vi "ConfigureDataEventCreator.vi"(8 "error in (no error)":errorcluster) -> (0 "error out":errorcluster, 2 "valid configuration":bool, 3 "config":T1)   [LabVIEW 2017, in "CmsDataEventCreator.lvlib"]
uses:
  <vilib>/addons/InsightCM/Devices/Shared/Cms/CmsDataEventCreator/CmsDataEventCreator.lvlib
  <vilib>/addons/InsightCM/Devices/Shared/Cms/CmsDataEventCreator/controls/config.ctl
  <vilib>/addons/InsightCM/Devices/Shared/Cms/CmsDataEventCreator/controls/DataEventConfig.ctl
  <vilib>/addons/InsightCM/Devices/Shared/Cms/CmsDataEventCreator/controls/AcqParams.ctl
  <vilib>/addons/InsightCM/Devices/Shared/Common/DataAccumulator/controls/AccumulationSettings.ctl
  <vilib>/addons/InsightCM/Devices/Shared/Common/DataAccumulator/controls/accumulationType.ctl
  <vilib>/addons/InsightCM/Devices/Shared/Common/DVRBuffer/controls/BufferLocation.ctl
  <vilib>/addons/PointValueMap/controls/PointMap.ctl
  <vilib>/addons/InsightCM/Devices/Shared/Cms/CmsDataEventCreator/controls/GroupRegistry.ctl
  <vilib>/addons/InsightCM/Devices/Shared/Cms/CmsDataEventCreator/controls/DataSetRegistry.ctl
  <vilib>/addons/InsightCM/Devices/Shared/Common/DataEvent/controls/DataSetType.ctl
  <vilib>/addons/InsightCM/Devices/Shared/Common/DataEventCreator/controls/Registry_Trend.ctl
  <vilib>/addons/InsightCM/Devices/Shared/Common/DataEvent/controls/Event.ctl
  <vilib>/addons/InsightCM/MessageBus/Base/controls/DataEvent.ctl
  <vilib>/addons/InsightCM/MessageBus/Base/controls/KeyValuePair.ctl
  <vilib>/addons/InsightCM/Devices/Shared/Common/DataEvent/controls/DataSet.ctl
  <vilib>/addons/InsightCM/MessageBus/Base/controls/DataSetMetadata.ctl
  <vilib>/addons/InsightCM/MessageBus/Base/controls/TrendPoint.ctl
  <vilib>/addons/InsightCM/MessageBus/Base/controls/TrendAlarmUpdate.ctl
  <vilib>/addons/InsightCM/MessageBus/Base/controls/TrendAlarmTransition.ctl
  <vilib>/addons/InsightCM/Utilities/GlobalConfiguration/GlobalConfiguration.lvlib
  <vilib>/addons/PointValueMap/PointValueMap.lvlib
  <vilib>/addons/InsightCM/Devices/Shared/Common/DataEvent/DataEvent.lvlib
  <vilib>/addons/InsightCM/Devices/Shared/Common/DataEventCreator/DataEventCreator.lvlib
  <vilib>/addons/InsightCM/Utilities/PropertyHelpers/PropertyHelpers.lvlib
  <vilib>/addons/InsightCM/Devices/Shared/Common/DVRBuffer/DVRBuffer.lvlib
  <vilib>/addons/InsightCM/Devices/Shared/Common/DataAccumulator/DataAccumulator.lvlib
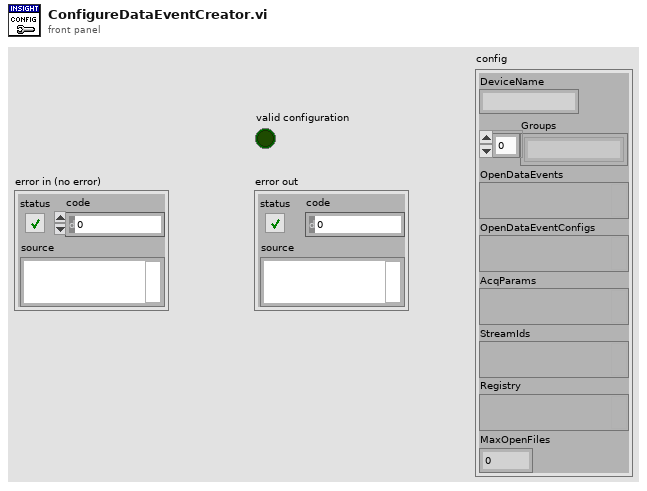
[diagram p1: front panel]
types:
  T1 = typedef "CmsDataEventCreator.lvlib/config.ctl" = cluster{"DeviceName":string, "Groups":string[], "OpenDataEvents":variant, "OpenDataEventConfigs":variant, "AcqParams":variant, "StreamIds":variant, "Registry":variant, "MaxOpenFiles":i32}
  T2 = typedef "SectionKeyValues.ctl" = cluster{"Section":string, "KeyValues":T3[]}
  T3 = typedef "KeyValuePair.ctl" = cluster{"Key":string, "Value":string}
  T4 = typedef "R2_Channel.ctl" = cluster{"Id":string, "DeviceId":string, "Name":string, "ChannelType":string, "HardwareKey":string, "HardwareChannel":string, "DataGroup":string, "Keywords":string[], "EquipmentIds":string[], "Properties":T3[], "Metrics":T5[], "AssetNodeId":string, "MeasType":string, "AssetName":string}
  T5 = typedef "Metric.ctl" = cluster{"Id":string, "Name":string, "Unit":string, "Properties":T3[], "MetricDefinitionInstanceId":string}
  T6 = typedef "R2_Device.ctl" = cluster{"Id":string, "Name":string, "DeviceType":string, "HardwareName":string, "IpAddress":string, "HardwareInfo":T3[], "ApplicationType":string, "ApplicationVersion":string, "EquipmentIds":string[], "ConfigurationVersion":string, "State":T7, "Properties":T3[], "DataGroups":T8[], "BurstModeTrigger":T12}
  T7 = typedef "DeviceState.ctl" = cluster{"Disabled":bool}
  T8 = typedef "R2_DataGroup.ctl" = cluster{"Name":string, "OperatingStates":T9[], "Properties":T3[], "EquipmentIds":string[], "AssetNodeId":string}
  T9 = typedef "OperatingState.ctl" = cluster{"Name":string, "Properties":T3[], "Triggers":T10[]}
  T10 = typedef "Trigger.ctl" = cluster{"Type":string, "Expression":string, "Conditions":T11[]}
  T11 = typedef "Condition.ctl" = cluster{"Source":string, "Type":string, "Operator":string, "CompareTo":string, "DwellSeconds":dbl}
  T12 = typedef "BurstModeTrigger.ctl" = cluster{"Trigger":T10, "SampleRate":string, "AcquisitionLength":string}
  T13 = typedef "DataEvent.lvlib/Event.ctl" = cluster{"DataEvent":T14, "DataSets":T15[], "TrendPoints":T17[], "Alarms":T18[]}
  T14 = typedef "DataEvent.ctl" = cluster{"Id":string, "AssetNodeId":string, "Timestamp":i64, "Props":T3[]}
  T15 = typedef "DataEvent.lvlib/DataSet.ctl" = cluster{"DataSetMetadata":T16, "Values":sgl[], "Values DVR":refnum<data-value>}
  T16 = typedef "DataSetMetadata.ctl" = cluster{"Id":string, "DataEventId":string, "AssetNodeId":string, "Type":string, "T0":i64, "Props":T3[]}
  T17 = typedef "TrendPoint.ctl" = cluster{"TrendPointId":string, "DataEventId":string, "Timestamp":i64, "Value":dbl, "Props":T3[]}
  T18 = typedef "TrendAlarmUpdate.ctl" = cluster{"RuleId":string, "Transition":T19}
  T19 = typedef "TrendAlarmTransition.ctl" = cluster{"At":i64, "Severity":i32, "Value":dbl, "Properties":T3[]}
  T20 = typedef "CmsDataEventCreator.lvlib/GroupRegistry.ctl" = cluster{"AssetNodeMap":variant, "DataSets":T21[], "Trends":T23[]}
  T21 = typedef "CmsDataEventCreator.lvlib/DataSetRegistry.ctl" = cluster{"ChannelName":string, "DataSetType":T22, "DoNotWriteToDB":bool, "ParentName":string, "CalculateOnServer":bool}
  T22 = typedef "DataEvent.lvlib/DataSetType.ctl" = enum16{"Waveform", "SpeedProfile", "ThermalImage", "EmsaSweep"}
  T23 = typedef "DataEventCreator.lvlib/Registry_Trend.ctl" = cluster{"TrendPointId":string, "DataSetName":string, "HighRate":bool, "Always Send":bool}
  T24 = typedef "CmsDataEventCreator.lvlib/DataEventConfig.ctl" = cluster{"AcqParams":T25, "OpState":string, "ExitOpState":bool, "Reason":string, "StreamId":string, "Map":T29, "DataSetIds":variant, "IncludeWaveforms":bool, "TrendPointsOnly":bool}
  T25 = typedef "CmsDataEventCreator.lvlib/AcqParams.ctl" = cluster{"Stream":bool, "PreTrigger":i32, "CollectOnEnter":bool, "Enter PreTrigger":i32, "Enter Length":dbl, "CollectOnExit":bool, "ContinuousData":bool, "Accumulation Settings":T26}
  T26 = typedef "DataAccumulator.lvlib/AccumulationSettings.ctl" = cluster{"Type":T27, "Length":dbl, "Max Time (sec)":dbl, "Start Block":T28, "Acquired (sec)":dbl, "Acquired (pulses)":i32, "Initial Pulse Offset":dbl, "Stop Block":T28, "LastBlockAdded":u32}
  T27 = typedef "DataAccumulator.lvlib/accumulationType.ctl" = enum16{"none", "seconds", "revolutions"}
  T28 = typedef "DVRBuffer.lvlib/BufferLocation.ctl" = cluster{"Block":u32, "Index":i32}
  T29 = typedef "PointValueMap.lvlib/PointMap.ctl" = refnum<data-value>
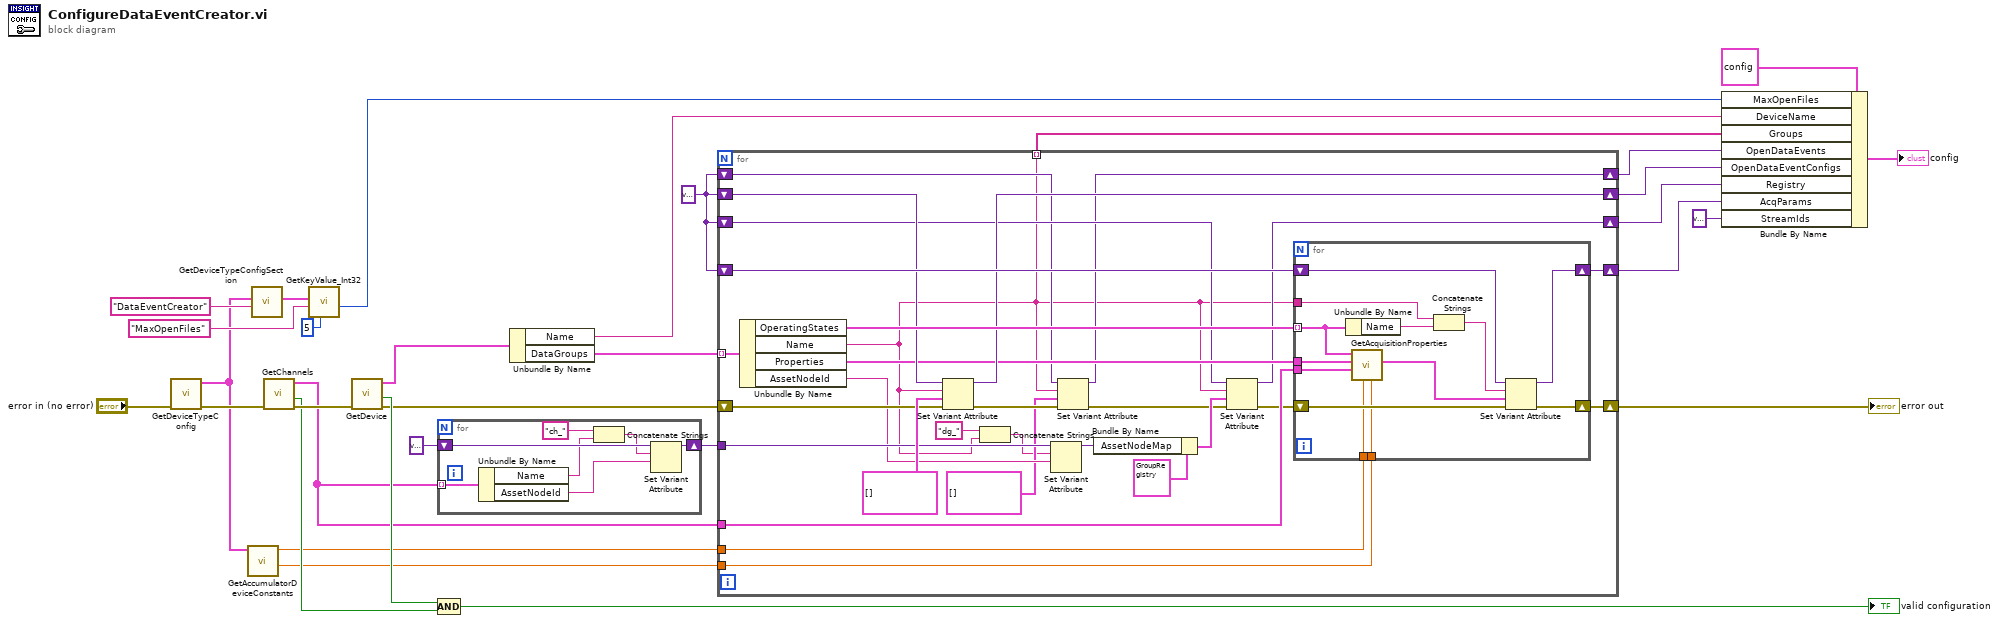
[diagram p0: block diagram]
diagram:
  w3 = variant
  n1 = call <vilib>:"GetDeviceTypeConfig.vi"("error in (no error)"="error in (no error)") -> ("error out"=w15:errorcluster, "key values"=w9:T2[])  [unwired: 8 in, 1 out]
  n2 = call <vilib>:"GetAccumulatorDeviceConstants.vi"("key values"=w9) -> ("default data block length (sec)"=w8:dbl, "max block (sec)"=w6:dbl)  [unwired: 6 in, 3 out]
  n3 = call <vilib>:"GetDeviceTypeConfigSection.vi"("key"="DataEventCreator", "key values"=w9) -> ("key value pairs out"=w13:T3[])  [unwired: 8 in, 1 out]
  n4 = call <vilib>:"GetChannels.vi"("error in (no error)"=w15) -> ("error out"=w23:errorcluster, "found"=w22:bool, "channels"=w18:T4[])  [unwired: 8 in]
  n5 = call <vilib>:"GetKeyValue_Int32.vi"("default"=5, "key"="MaxOpenFiles", "key value pairs"=w13) -> ("value"=w10:i32)  [unwired: 6 in, 2 out]
  n6 = call <vilib>:"GetDevice.vi"("error in (no error)"=w23) -> ("error out"=w20:errorcluster, "found"=w27:bool, "device configuration"=w30:T6)  [unwired: 8 in]
  n7 = for {
    shift-right: [w36] -> w17
    shift-left: variant -> [w37]
    tunnel: w18 -> [w38] mode=indexing
    n8 = Unbundle By Name(w38) -> ("Name"=w33:string, "AssetNodeId"=w35:string)
    n9 = Concatenate Strings("ch_" ("string"), w33) -> (w32:string)
    n10 = Set Variant Attribute(Variant=w37, name=w32, value=w35) -> (Variant out=w36:variant)  [unwired: 1 in, 2 out]
  }
  n11 = Compound Arithmetic op=AND(w27, w22) -> (→"valid configuration":bool)
  n12 = Unbundle By Name(w30) -> ("Name"=w24:string, "DataGroups"=w31:T8[])
  n13 = for {
    shift-right: [w56] -> w29
    shift-left: w20 -> [w57]
    tunnel: w31 -> [w66] mode=indexing
    shift-right: [w63] -> w25
    shift-left: w3 -> [w65]
    shift-right: [w61] -> w4
    shift-left: w3 -> [w62]
    tunnel: w18 -> [w58]
    shift-right: [w54] -> w5
    shift-left: w3 -> [w55]
    tunnel: w17 -> [w50]
    tunnel: w8 -> [w48]
    tunnel: w6 -> [w47]
    shift-right: [w43] -> w2
    shift-left: w3 -> [w44]
    tunnel: [w39] -> w1 mode=indexing
    n14 = Unbundle By Name(w66) -> ("OperatingStates"=w64:T9[], "Name"=w39:string, "Properties"=w59:T3[], "AssetNodeId"=w49:string)
    n15 = Set Variant Attribute(Variant=w62, name=w39, value=T24[] [], error in=w57) -> (Variant out=w61:variant, error out=w46:errorcluster)  [unwired: 1 out]
    n16 = Concatenate Strings("dg_" ("string"), w39) -> (w40:string)
    n17 = Set Variant Attribute(Variant=w50, name=w40, value=w49) -> (Variant out=w51:variant)  [unwired: 1 in, 2 out]
    n18 = Set Variant Attribute(Variant=w44, name=w39, value=T13[] [] ("data events"), error in=w46) -> (Variant out=w43:variant, error out=w45:errorcluster)  [unwired: 1 out]
    n19 = Bundle By Name(cluster=T20 {"AssetNodeMap"=variant, "DataSets"=[], "Trends"=[]} ("Data Group Registry"), "AssetNodeMap"=w51) -> (w52:T20)
    n20 = Set Variant Attribute(Variant=w55, name=w39, value=w52, error in=w45) -> (Variant out=w54:variant, error out=w56:errorcluster)  [unwired: 1 out]
    n21 = for {
      shift-right: [w69] -> _
      shift-left: w56 -> [w79]
      shift-right: [w77] -> w63
      shift-left: w65 -> [w78]
      tunnel: w39 -> [w75]
      tunnel: w64 -> [w73] mode=indexing
      tunnel: w59 -> [w72]
      tunnel: w58 -> [w71]
      tunnel: w48 -> [w67]
      tunnel: w47 -> [w68]
      n22 = Unbundle By Name(w73) -> ("Name"=w76:string)
      n23 = call <vilib>:"GetAcquisitionProperties.vi"("default data block length"=w67, "max time (sec)"=w68, "channels"=w71, "group properties"=w72, "operating state"=w73) -> ("AcqParams"=w70:T25)  [unwired: 6 in]
      n24 = Concatenate Strings(w75, w76) -> (w74:string)
      n25 = Set Variant Attribute(Variant=w78, name=w74, value=w70, error in=w79) -> (Variant out=w77:variant, error out=w69:errorcluster)  [unwired: 1 out]
    }
  }
  "error out" <- w29
  n26 = Bundle By Name(cluster=T1 {"DeviceName"="", "Groups"=[], "OpenDataEvents"=variant, "OpenDataEventConfigs"=variant, "AcqParams"=variant, "StreamIds"=variant, "Registry"=variant, "MaxOpenFiles"=0} ("config"), "MaxOpenFiles"=w10, "DeviceName"=w24, "Groups"=w1, "OpenDataEvents"=w2, "OpenDataEventConfigs"=w4, "Registry"=w5, "AcqParams"=w25, "StreamIds"=variant ("OpStateCorrId")) -> (→"config":T1)
